vi "RegisterCEPMLocalFeed.vi"(8 "Error In":errorcluster) -> (0 "Error Out":errorcluster)   [LabVIEW 2019, in "CEPM.lvlib"]
uses:
  CEPM.lvlib
  <vilib>/National Instruments/NIPM API (Beta)/NIPM_API.lvlib
  <vilib>/SLL Toolkit/SLL File IO/SLL File IO.lvlib
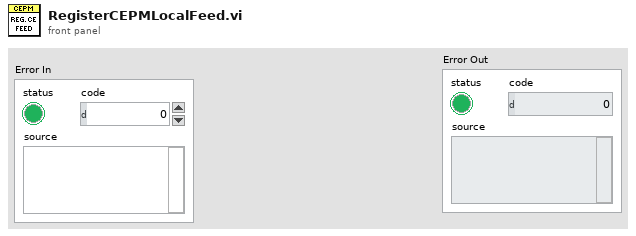
[diagram p1: front panel]
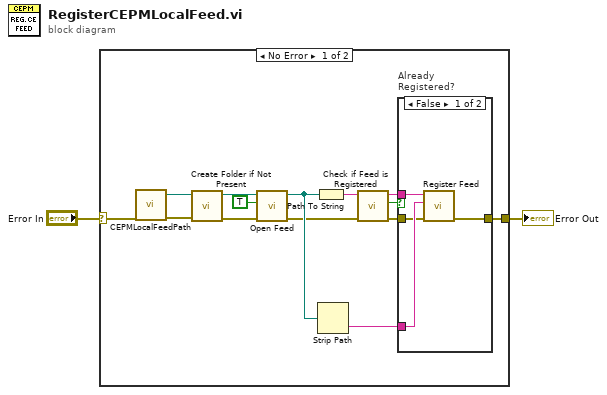
[diagram p0: block diagram]
diagram:
  n1 = case shown="No Error" "Error In" {
    selector: "Error In" -> [w12 w22]
    tunnel: [w16 w22] -> w1
    frame No Error {
      n2 = call "CEPMLocalFeedPath.vi"("Error In"=w12) -> ("Error Out"=w11:errorcluster, "CEPM Local Feed Path"=w10:path)  [unwired: 9 in]
      n3 = call <vilib>:"Create Folder if Not Present.vi"("error in (no error)"=w11, "Path"=w10) -> ("error out"=w15:errorcluster, "Path out"=w14:path)  [unwired: 8 in]
      n4 = call <vilib>:"Open Feed.vi"("error in"=w15, "create feed if necessary (F)"=TRUE, "feed folderpath"=w14) -> ("error out"=w7:errorcluster, "feed folderpath out"=w9:path)  [unwired: 6 in, 1 out]
      n5 = Path To String(path=w9) -> (string=w6:string)
      n6 = Strip Path(path=w9) -> (name=w8:string)  [unwired: 1 out]
      n7 = call <vilib>:"Check if Feed is Registered.vi"("error in"=w7, "feed URI"=w6) -> ("error out"=w4:errorcluster, "feed URI registered?"=w3:bool, "feed URI out"=w5:string)  [unwired: 6 in, 1 out]
      n8 = case "Already \nRegistered?" shown="False" w3 {
        tunnel: [w20 w21] -> w16
        tunnel: w8 -> [w19 _]
        tunnel: w5 -> [w18 _]
        tunnel: w4 -> [w17 w21]
        frame False {
          n9 = call <vilib>:"Register Feed.vi"("error in"=w17, "feed name"=w19, "feed URI"=w18) -> ("error out"=w20:errorcluster)  [unwired: 7 in, 1 out]
        }
        frame True {
        }
      }
    }
    frame Error {
    }
  }
  "Error Out" <- w1
